vi "Read Session Refnum.vi"(8 "error in (no error)":errorcluster, 11 "session":T4) -> (0 "error out":errorcluster, 1 "abstract":T3, 2 "LIBSSH2_SESSION*":u64, 3 "semaphore":T1, 4 "events":T2)   [LabVIEW 2017, in "libssh2.lvlib"]
uses:
  libssh2.lvlib
  Session Refnum.ctl
  libssh2_session_abstract.ctl
  lvssh2_session_callback_events.ctl
  lvssh2_session_callback_send_function_input_args_32.ctl
  lvssh2_session_callback_receive_function_input_args_32.ctl
  lvssh2_userauth_keyboard_interactive_response_function_input_args_32.ctl
  lvssh2_session_callback_send_function_input_args_64.ctl
  lvssh2_session_callback_receive_function_input_args_64.ctl
  lvssh2_userauth_keyboard_interactive_response_function_input_args_64.ctl
  Session Refnum Data.ctl
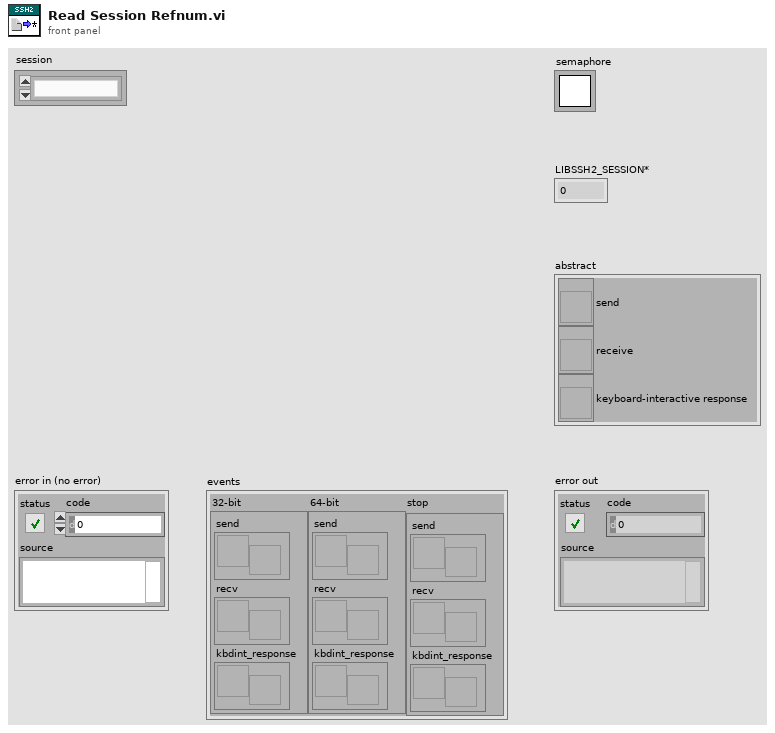
[diagram p1: front panel]
types:
  T1 = typedef "Semaphore RefNum" = refnum<k1>
  T2 = typedef "libssh2.lvlib/lvssh2_session_callback_events.ctl" = cluster{"32-bit":cluster{"send":refnum<user-event>, "recv":refnum<user-event>, "kbdint_response":refnum<user-event>}, "64-bit":cluster{"send":refnum<user-event>, "recv":refnum<user-event>, "kbdint_response":refnum<user-event>}, "stop":cluster{"send":refnum<user-event>, "recv":refnum<user-event>, "kbdint_response":refnum<user-event>}}
  T3 = typedef "libssh2.lvlib/libssh2_session_abstract.ctl" = cluster{"send":refnum<vi>, "receive":refnum<vi>, "keyboard-interactive response":refnum<vi>}
  T4 = typedef "libssh2.lvlib/Session Refnum.ctl" = refnum<k1>
  T5 = typedef "libssh2.lvlib/Session Refnum Data.ctl" = cluster{"LIBSSH2_SESSION*":u64, "abstract":T3, "events":T2, "semaphore":T1}
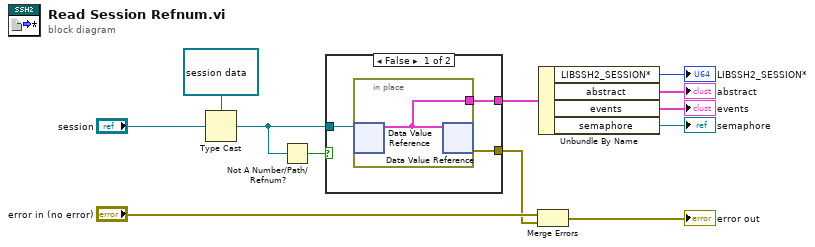
[diagram p0: block diagram]
diagram:
  n1 = Type Cast(type=refnum<data-value> refnum ("data value reference"), x="session") -> (*(type *) &x=w7:refnum<data-value>)
  n2 = Not A Number/Path/Refnum?(number/path/refnum=w7) -> (NaN/Path/Refnum?=w6:bool)
  n3 = case shown="False" w6 {
    tunnel: w7 -> [w15 _]
    tunnel: [w14 _] -> w11
    tunnel: [w13 _] -> w8
    frame False {
      n4 = in-place {
        in-place-border: [w16] -> w14
        n5 = in-place-dvr #1(w15) -> (w16:T5)  [unwired: 1 out]
        n6 = in-place-dvr #1(w16) -> (w13:errorcluster)  [unwired: 1 out]
      }
    }
    frame True {
    }
  }
  n7 = Merge Errors("error in (no error)", w8) -> (→"error out":errorcluster)
  n8 = Unbundle By Name(w11) -> ("LIBSSH2_SESSION*"=→"LIBSSH2_SESSION*":u64, "abstract"=→"abstract":T3, "events"=→"events":T2, "semaphore"=→"semaphore":T1)
